vi "Wait till limit reached.vi"(8 "error in (no error)":errorcluster, 10 "Axis Number":i32, 11 ".NET Refnum in":T1) -> (0 "error out":errorcluster, 3 ".NET Refnum out":T1)   [LabVIEW 2016, in "Drivers.lvlib" / "Agilis.lvlib"]
uses:
  Agilis.lvlib
  AgilisCmdLib Refnum.ctl
  D:/Trace Grabber/Drivers/Agilis/AgilisCmdLib.dll
  AgilisCmdLib.dll
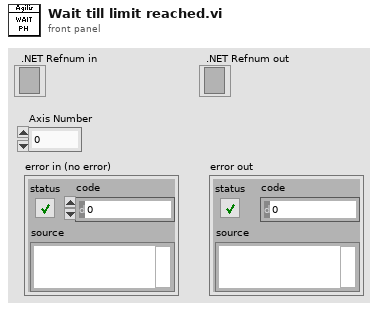
[diagram p1: front panel]
types:
  T1 = typedef "Drivers.lvlib/Agilis.lvlib/AgilisCmdLib Refnum.ctl" = refnum<k24>
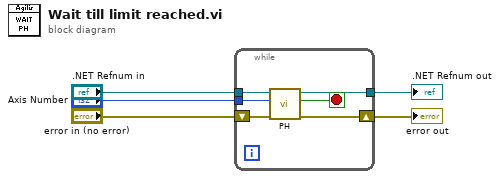
[diagram p0: block diagram]
diagram:
  n1 = while {
    tunnel: ".NET Refnum in" -> [w10]
    tunnel: [w9] -> w5
    shift-right: [w8] -> w4
    shift-left: "error in (no error)" -> [w11]
    tunnel: "Axis Number" -> [w7]
    stop <- w6 stop-if-true
    n2 = call "PH.vi"("error in (no error)"=w11, "Axis Number"=w7, "Agilis in"=w10) -> ("error out"=w8:errorcluster, "Triggered?"=w6:bool, "Agilis out"=w9:T1)  [unwired: 5 in, 1 out]
  }
  "error out" <- w4
  ".NET Refnum out" <- w5
